vi "Set Channel Enable Analog Out.vi"(7 "fEnable":bool=TRUE, 8 "error in (no error)":errorcluster, 9 "node":T1, 10 "idxChannel":i32, 11 "hdwf":i32) -> (0 "error out":errorcluster)   [LabVIEW 2014, in "AnalogDiscSDKLv.lvlib"]
doc: "extern \"C\" __declspec(dllexport) int SetChannelEnable_AnalogOut(\n HDWF hdwf,\n int idxChannel,\n AnalogOutNode node,\n int fEnable\n );"
uses:
  <instrlib>/AnalogDiscSDKLv/AnalogDiscSDKLv.lvlib
  <instrlib>/AnalogDiscSDKLv/VIs/DWF_Node.ctl
  <instrlib>/AnalogDiscSDKLv/AnalogDiscSDKLv.dll
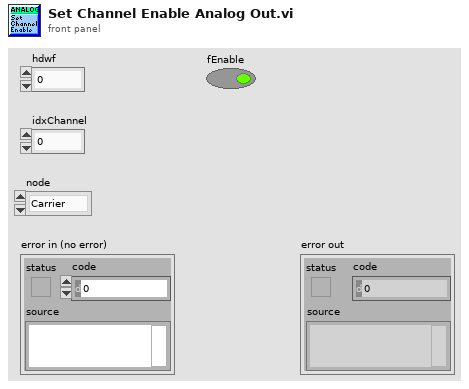
[diagram p1: front panel]
types:
  T1 = typedef "AnalogDiscSDKLv.lvlib/DWF_Node.ctl" = enum16{"Carrier", "FM", "AM"}
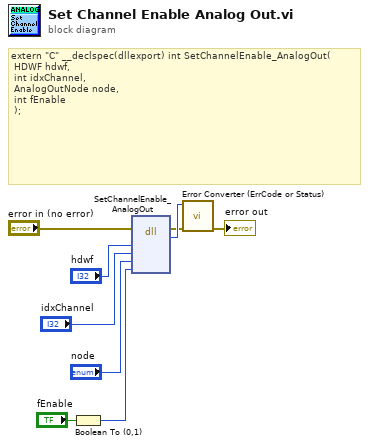
[diagram p0: block diagram]
diagram:
  # "extern \"C\" __declspec(dllexport) int SetChannelEnable_AnalogOut(\n\tHDWF hdwf,\n\tint idxChannel,\n\tAnalogOutNode node,\n\tint fEnable\n\t);"
  n1 = Boolean To (0,1)(Boolean="fEnable") -> (0, 1=w1:i16)
  n2 = dll-call lib="C:/Program Files (x86)/National Instruments/LabVIEW 2014/instr.lib/AnalogDiscSDKLv/AnalogDiscSDKLv.*" fn="SetChannelEnable_AnalogOut"(error in="error in (no error)", "hdwf"="hdwf", "idxChannel"="idxChannel", "node"="node", "fEnable"=w1) -> (error out=w3:errorcluster, w4:i32)  [unwired: 6 in, 1 out]
  n3 = call <instrlib>:"Error Converter (ErrCode or Status).vi"("error in (no error)"=w3, "error code"=w4) -> ("error out"=→"error out":errorcluster)  [unwired: 9 in]
